vi "setFPGAReference.vi"(10 "FPGAReference":refnum<k20>, 11 "MockDisplacementCommandFIFO in":refnum<class "MockDisplacementlCommandFIFO.lvclass">) -> (3 "MockDisplacementCommandFIFO out":refnum<class "MockDisplacementlCommandFIFO.lvclass">)   [LabVIEW 2016, in "MockDisplacementlCommandFIFO.lvclass"]
uses:
  MockDisplacementlCommandFIFO.lvclass
  MockDisplacementlCommandFIFO.lvclass/MockDisplacementlCommandFIFO.ctl
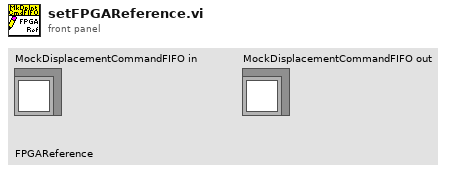
[diagram p1: front panel]
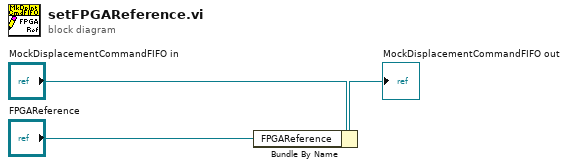
[diagram p0: block diagram]
diagram:
  n1 = Bundle By Name(cluster="MockDisplacementCommandFIFO in", "FPGAReference"="FPGAReference") -> (→"MockDisplacementCommandFIFO out":refnum<class "MockDisplacementlCommandFIFO.lvclass">)
